vi "Open.vi"(8 "error in (no error)":errorcluster, 11 "MelsecTCP in":refnum<class "ModbusRtu.lvclass">) -> (0 "error out":errorcluster, 3 "MelsecTCP out":refnum<class "ModbusRtu.lvclass">)   [LabVIEW 2020, in "HslCommunication.lvlib" / "ModbusRtu.lvclass"]
uses:
  ModbusRtu.lvclass
  ModbusRtu.lvclass/ModbusRtu.ctl
  E:/Git/Libraries/develop/HslCommunication/_Dependenciecs/HslCommunication.dll
  _Dependenciecs/HslCommunication.dll
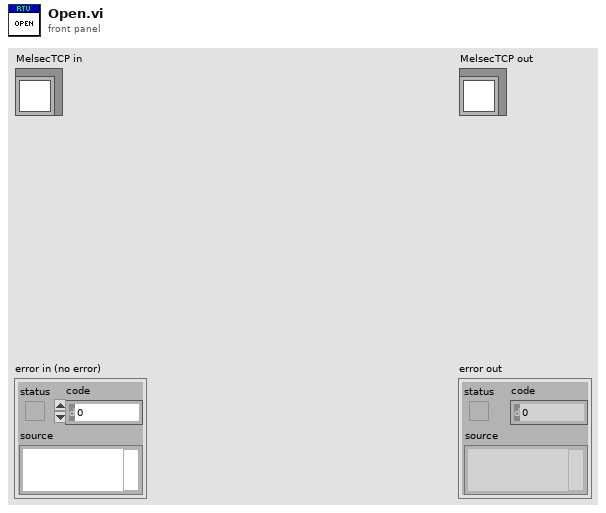
[diagram p1: front panel]
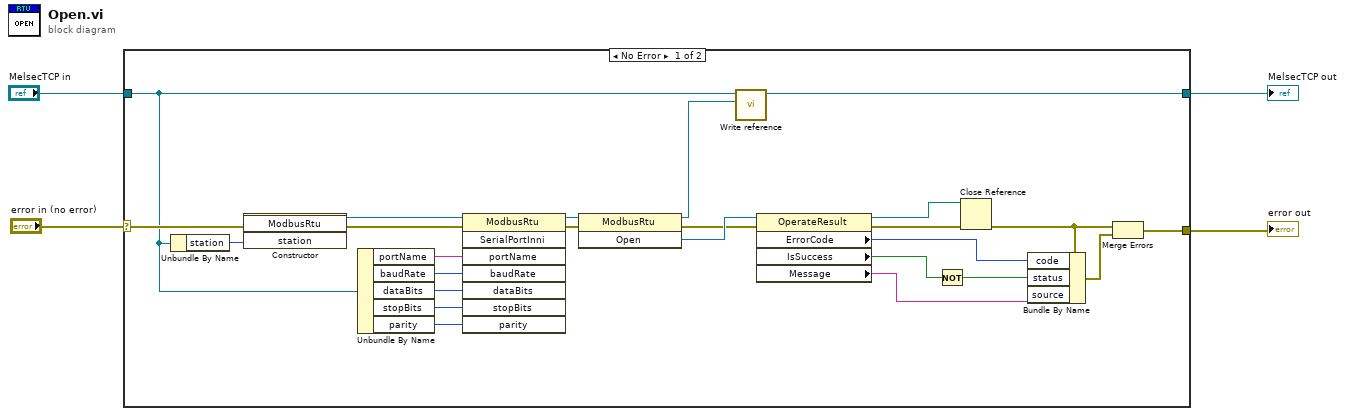
[diagram p0: block diagram]
diagram:
  n1 = case shown="No Error" "error in (no error)" {
    selector: "error in (no error)" -> [w19 w31]
    tunnel: "MelsecTCP in" -> [w9 w30]
    tunnel: [w6 w30] -> w1
    tunnel: [w25 w31] -> w2
    frame No Error {
      n2 = Unbundle By Name(w9) -> ("station"=w10:u8)
      n3 = constructor class="ModbusRtu"(error in=w19, "station"=w10) -> (reference out=w7:refnum<k24>, error out=w22:errorcluster)  [unwired: 2 in, 2 out]
      n4 = Unbundle By Name(w9) -> ("portName"=w11:string, "baudRate"=w15:i32, "dataBits"=w14:i32, "stopBits"=w13:i32, "parity"=w12:i32)
      n5 = invoke class="ModbusRtu" method="SerialPortInni"(reference=w7, error in=w22, "portName"=w11, "baudRate"=w15, "dataBits"=w14, "stopBits"=w13, "parity"=w12) -> (reference out=w20:refnum<k24>, error out=w18:errorcluster)  [unwired: 1 in, 6 out]
      n6 = invoke class="ModbusRtu" method="Open"(reference=w20, error in=w18) -> (reference out=w5:refnum<k24>, error out=w16:errorcluster, "Open"=w17:refnum<k24>)  [unwired: 1 in]
      n7 = call-dynamic "Write reference.vi"("reference"=w5, "MelsecTCP in"=w9) -> ("MelsecTCP out"=w6:refnum<class "ModbusRtu.lvclass">)  [unwired: 8 in, 1 out]
      n8 = property class="OperateResult"(reference=w17, error in=w16) -> (reference out=w24:refnum<k24>, error out=w23:errorcluster, "ErrorCode"=w28:i32, "IsSuccess"=w21:bool, "Message"=w26:string)
      n9 = Not(x=w21) -> (.not. x?=w27:bool)
      n10 = Close Reference(reference=w24, error in (no error)=w23) -> (error out=w8:errorcluster)
      n11 = Bundle By Name(cluster=w8, "code"=w28, "status"=w27, "source"=w26) -> (w29:errorcluster)
      n12 = Merge Errors(w8, w29) -> (w25:errorcluster)
    }
    frame Error {
    }
  }
  "error out" <- w2
  "MelsecTCP out" <- w1
